vi "Table Value To 1D DBL Without Exception Number.vi"(8 "End Number":dbl=nan, 9 "Exception Number":dbl=-1.0, 11 "Table Ref In":refnum<vi>) -> (1 "DBL Out":dbl[](array[numeric]), 3 "Table Ref Out":refnum<vi>)   [LabVIEW 2024]
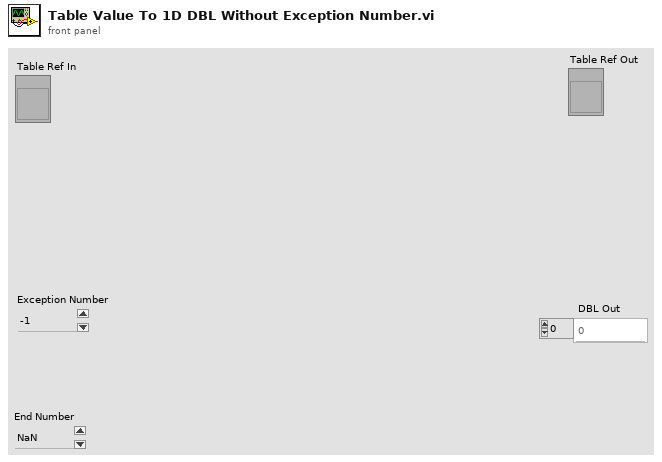
[diagram p1: front panel]
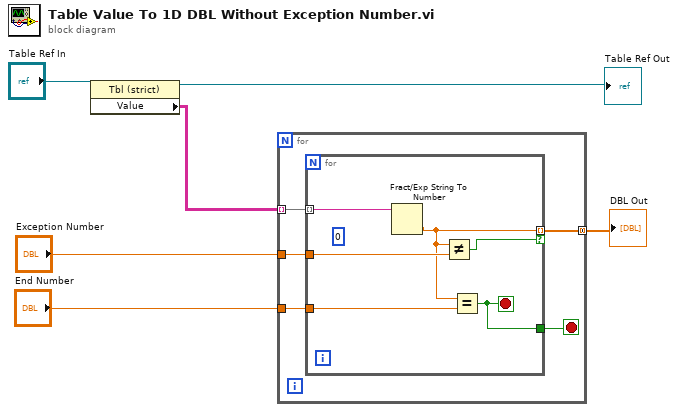
[diagram p0: block diagram]
diagram:
  n1 = property class="Tbl (strict)"(reference="Table Ref In") -> (reference out=→"Table Ref Out":refnum<vi>, "Value"=w4:string[][])  [unwired: 1 in, 1 out]
  n2 = for {
    tunnel: w4 -> [w11] mode=indexing
    tunnel: "Exception Number" -> [w10]
    tunnel: [w9] -> w2 mode=concatenating
    tunnel: "End Number" -> [w8]
    stop <- w7 stop-if-true
    n3 = for {
      tunnel: w11 -> [w13] mode=indexing
      tunnel: [w12] -> w9 mode=indexing if=w17
      tunnel: w10 -> [w16]
      tunnel: w8 -> [w15]
      tunnel: [w14] -> w7
      stop <- w14 stop-if-true
      (unwired) i64 0 ("default (0 I32)")
      n4 = Fract/Exp String To Number(string=w13) -> (number=w12:dbl)  [unwired: 3 in, 1 out]
      n5 = Not Equal?(x=w12, y=w16) -> (x != y?=w17:bool)
      n6 = Equal?(x=w12, y=w15) -> (x = y?=w14:bool)
    }
  }
  "DBL Out" <- w2
